vi "borrar despues.vi"() -> ()   [LabVIEW 2019]
panel:
  in  "Simulacion":bool
  in  "Tipo de generador":string
  in  "Ruta de configuracion":path
  in  "Control references":T1(array[cluster])
  # "LeerArchivoConfiguracion"
  # "InicializarInstrumentos"
  # "DetieneInstrumentos"
  # "ConfirmarSalida"
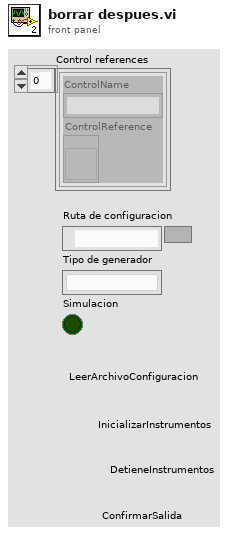
[diagram p1: front panel]
types:
  T1 = cluster{"ControlName":string, "ControlReference":refnum<vi>}[]
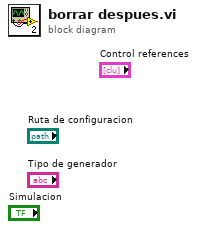
[diagram p0: block diagram]
diagram:
